vi "Duplicate Files.vi"(8 "error in (no error)":errorcluster, 10 "Number of Files":i32, 11 "path":path=path "C:/user/patrick/other/test/filename.itx") -> (0 "error out":errorcluster)   [LabVIEW 2016]
panel:
  in  "stop":bool
  out "Numeric":i32=5699
  out "x-y":u32=5
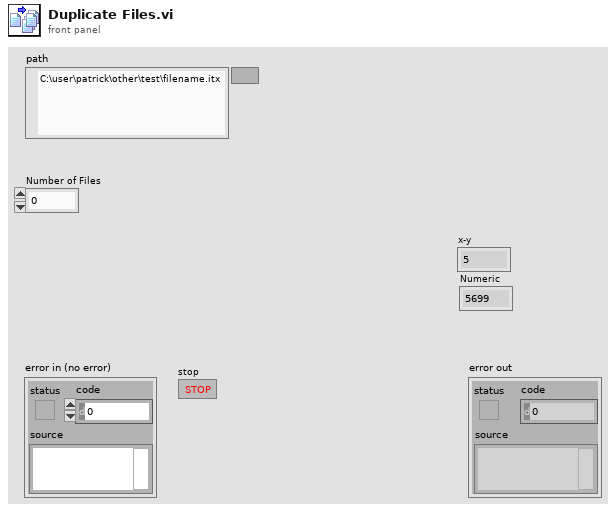
[diagram p1: front panel]
types:
  T1 = enum16{"open", "replace", "create", "open or create", "replace or create", "replace or create with confirmation"}
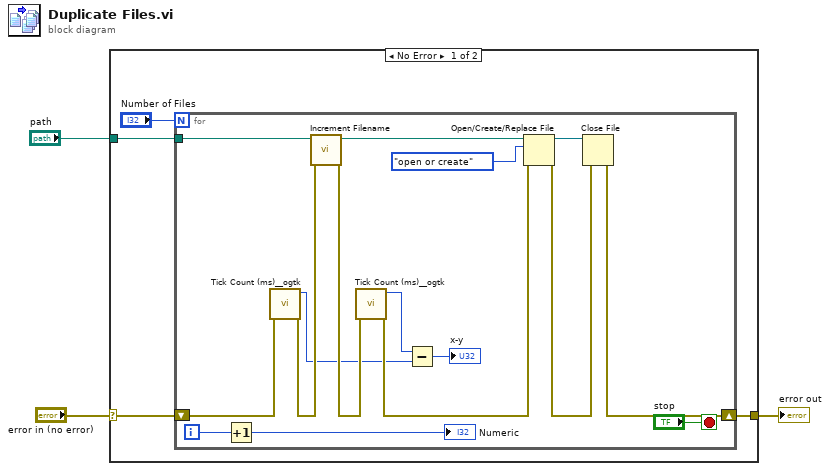
[diagram p0: block diagram]
diagram:
  n1 = case shown="No Error" "error in (no error)" {
    selector: "error in (no error)" -> [w7 w24]
    tunnel: [w6 w24] -> w2
    tunnel: "path" -> [w5 _]
    frame No Error {
      n2 = for {
        N: "Number of Files" -> [_]
        shift-right: [w20] -> w6
        shift-left: w7 -> [w18]
        tunnel: w5 -> [w9]
        i -> [w12]
        stop <- "stop" stop-if-true
        n3 = Increment(x=w12) -> (x+1=→"Numeric":i32)
        n4 = call "Tick Count (ms)__ogtk.vi"("error in (no error)"=w18) -> ("error out"=w19:errorcluster, "millisecond timer value"=w14:u32)  [unwired: 9 in]
        n5 = call "Increment Filename.vi"("error in (no error)"=w19, "Path"=w9) -> ("error out"=w17:errorcluster, "Modified Path"=w23:path)  [unwired: 8 in]
        n6 = call "Tick Count (ms)__ogtk.vi"("error in (no error)"=w17) -> ("error out"=w16:errorcluster, "millisecond timer value"=w15:u32)  [unwired: 9 in]
        n7 = Subtract(x=w15, y=w14) -> (x-y=→"x-y":u32)
        n8 = Open/Create/Replace File(file path (use dialog)=w23, error in=w16, operation (0:open)=T1."open or create") -> (refnum out=w21:refnum<file>, error out=w22:errorcluster)  [unwired: 3 in, 1 out]
        n9 = Close File(refnum=w21, error in=w22) -> (error out=w20:errorcluster)  [unwired: 1 out]
      }
    }
    frame Error {
    }
  }
  "error out" <- w2
